vi "James.vi"(8 "error in (no error)":errorcluster, 11 "module in":refnum<class>) -> (0 "error out":errorcluster, 3 "module out":refnum<class>)   [LabVIEW 2024]
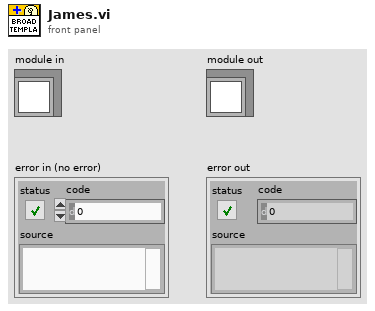
[diagram p1: front panel]
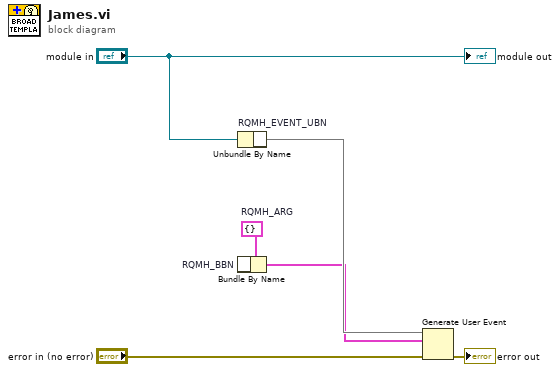
[diagram p0: block diagram]
diagram:
  w3 = cluster{} {}  # RQMH_ARG
  n1 = Unbundle By Name "RQMH_EVENT_UBN"("module in") -> (w6)
  n2 = Bundle By Name "RQMH_BBN"(cluster=w3) -> (w2:cluster{})  [unwired: 1 in]
  n3 = Generate User Event(user event=w6, event data cluster=w2, error in="error in (no error)") -> (error out=→"error out":errorcluster)  [unwired: 1 in, 1 out]
  "module out" <- "module in"
